vi "FTW-Connector-LaunchActor.vi"(0 "FTW Actor Connector Type":refnum<class "FTW-ActorConnector.lvclass">, 5 "Actor VI Filepath":path, 7 "Configuration":string, 11 "error in":errorcluster) -> (4 "FTW Actor Connector":refnum<class "FTW-ActorConnector.lvclass">, 15 "error out":errorcluster)   [LabVIEW 2013, in "FTW-Actor.lvlib" / "FTW-ActorConnector.lvclass"]
uses:
  FTW-ActorConnector.lvclass
  FTW-Actor.lvlib
  Core/utils/CodeGen/JSON Deserialize/FTW-JSON-Deserialize.xnode
  Core/src/Reflection/FTW-Reflection-Type.vi
  Core/src/JSON/FTW-JSON-Core-GetFlattenedValue.vi
  Core/src/JSON/FTW-JSON-Core-LibraryFilepath.vi
  Core/src/JSON/FTW-JSON-Core-LibraryError.vi
panel:
  # "Inputs"
  # "Outputs"
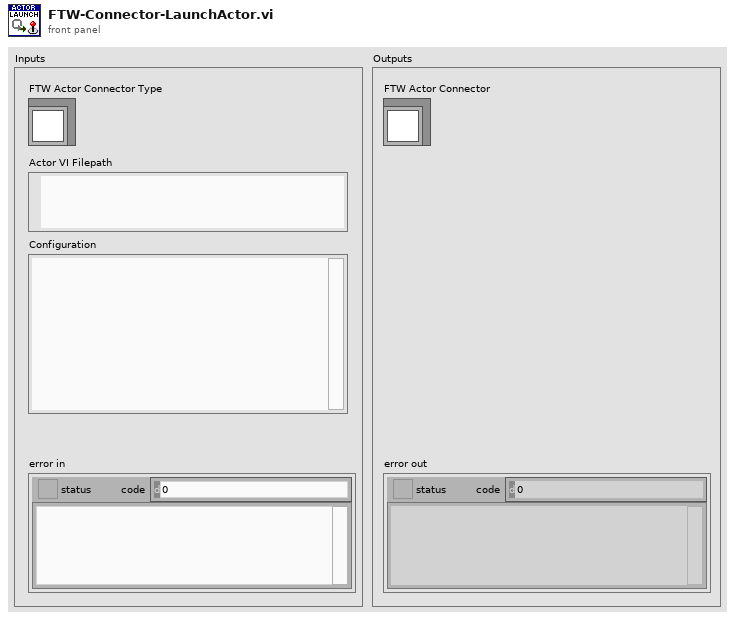
[diagram p1: front panel]
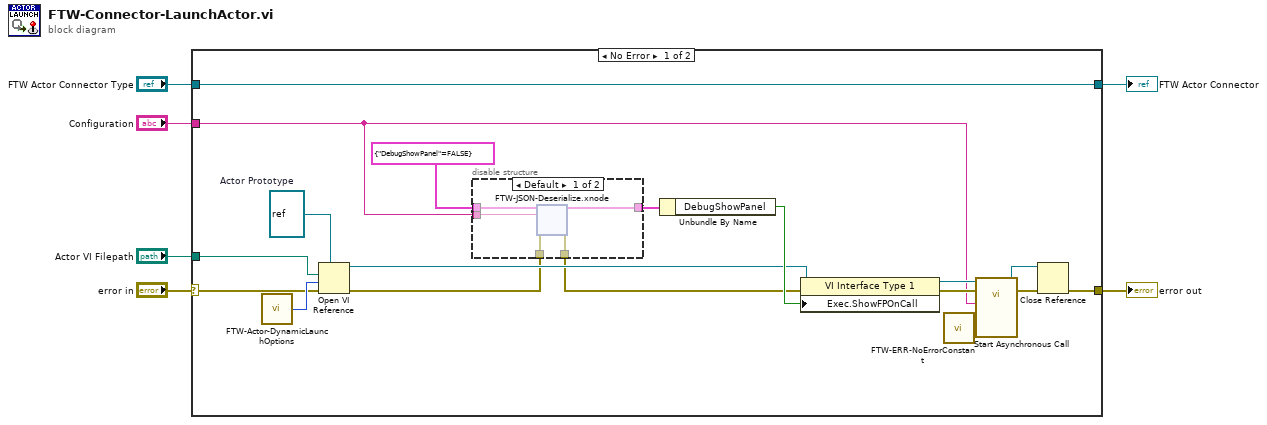
[diagram p0: block diagram]
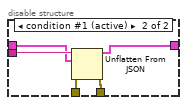
[diagram p2: hidden frame]
diagram:
  n1 = case shown="No Error" "error in" {
    selector: "error in" -> [w20 w70]
    tunnel: [w22 w70] -> w6
    tunnel: "Configuration" -> [w11 _]
    tunnel: [w21 w69] -> w3
    tunnel: "FTW Actor Connector Type" -> [w21 w69]
    tunnel: "Actor VI Filepath" -> [w19 _]
    frame No Error {
      w24 = refnum<vi> refnum  # Actor Prototype
      n2 = call "FTW-Actor-DynamicLaunchOptions.vi"() -> ("Open VI Ref Options"=w23:i32)
      n3 = Open VI Reference(type specifier VI Refnum (for type only)=w24, vi path=w19, options=w23, error in (no error)=w20) -> (vi reference=w12:refnum<vi>, error out=w10:errorcluster)  [unwired: 2 in]
      n4 = disable-structure shown="Default" {
        disable-tunnel: w11 -> [w29 w68]
        disable-tunnel: w10 -> [w28 w67]
        disable-tunnel: [w27 w66] -> w9
        disable-tunnel: [w26 w64] -> w8
        disable-tunnel: cluster{"DebugShowPanel":bool} {"DebugShowPanel"=FALSE} -> [w25 w65]
        frame condition #0 {
          n5 = xnode "FTW-JSON-Deserialize.xnode"("Type and Defaults"=w25, "JSON String"=w29, "error in"=w28) -> ("Values"=w26:cluster{"DebugShowPanel":bool}, "error out"=w27:errorcluster)
        }
        frame condition #1 (active) {
          n6 = Unflatten From JSON(JSON string=w68, type and defaults=w65, error in (no error)=w67) -> (value=w64:cluster{"DebugShowPanel":bool}, error out=w66:errorcluster)  [unwired: 4 in]
        }
      }
      n7 = Unbundle By Name(w8) -> ("DebugShowPanel"=w13:bool)
      n8 = property class="VI Interface Type 1"(reference=w12, error in=w9, "Exec.ShowFPOnCall"=w13) -> (reference out=w15:refnum<vi>, error out=w14:errorcluster)
      n9 = call "FTW-ERR-NoErrorConstant.vi"() -> ("no error"=w18:errorcluster)
      n10 = call-by-ref "Start Asynchronous Call"(reference=w15, error in=w14, "Configuration"=w11, "ErrorIn"=w18) -> (reference out=w17:refnum<vi>, error out=w16:errorcluster)  [unwired: 13 in, 1 out]
      n11 = Close Reference(reference=w17, error in (no error)=w16) -> (error out=w22:errorcluster)
    }
    frame Error {
    }
  }
  "error out" <- w6
  "FTW Actor Connector" <- w3
